vi "Schedule Update.vi"(8 "error in (no error)":errorcluster, 11 "Model in":refnum<class "Model.lvclass">) -> (0 "error out":errorcluster, 3 "Model out":refnum<class "Model.lvclass">)   [LabVIEW 2016, in "Model.lvclass"]
uses:
  Model.lvclass
  Typedefs/CommandTypes.ctl
  Model.lvclass/Model.ctl
  User Events/User Events.lvclass/User Events.ctl
  Commands/Command Factory/Command Factory.lvclass
  User Events/User Events.lvclass
  Typedefs/HPMT_Typedefs.lvlib
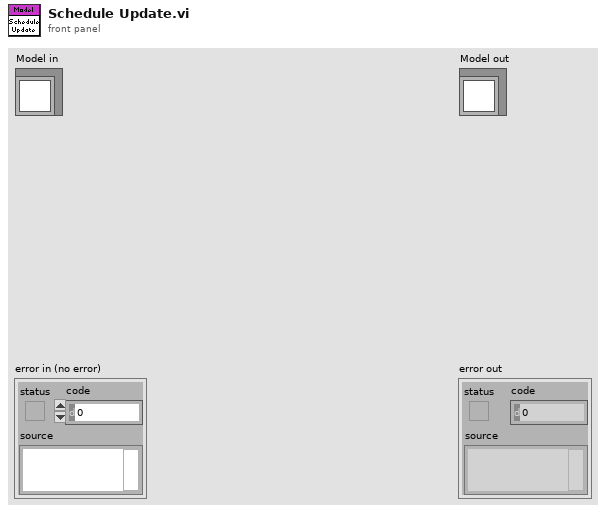
[diagram p1: front panel]
types:
  T1 = typedef "HPMT_Typedefs.lvlib/CommandTypes.ctl" = enum16{"Start", "Enable", "Disable", "Standby", "Shutdown", "Update"}
  T2 = typedef "HPMT_Typedefs.lvlib/Subscribe Data Events.ctl" = cluster{"Command":refnum<user-event>}
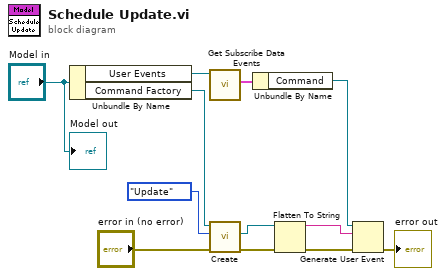
[diagram p0: block diagram]
diagram:
  n1 = Unbundle By Name("Model in") -> ("User Events"=w11:refnum<class "User Events.lvclass">, "Command Factory"=w9:refnum<class "Command Factory.lvclass">)
  n2 = call "Get Subscribe Data Events.vi"("UserEvents in"=w11) -> ("Subscribe Data Events"=w10:T2)  [unwired: 9 in, 1 out]
  n3 = call-dynamic "Create.vi"("error in (no error)"="error in (no error)", "Command Types"=CommandTypes."Update" ("Command"), "Command Factory in"=w9) -> ("error out"=w3:errorcluster, "Command"=w7:refnum<class "Command.lvclass">)  [unwired: 6 in, 1 out]
  n4 = Unbundle By Name(w10) -> ("Command"=w5:refnum<user-event>)
  n5 = Flatten To String(anything=w7, error in (no error)=w3) -> (data string=w6:string, error out=w2:errorcluster)  [unwired: 2 in, 1 out]
  n6 = Generate User Event(user event=w5, event data cluster=w6, error in=w2) -> (error out=→"error out":errorcluster)  [unwired: 1 in, 1 out]
  "Model out" <- "Model in"
